vi "HexStringToBoolean.vi"(1 "Hex String":string) -> (0 "Boolean":bool)   [LabVIEW 2023]
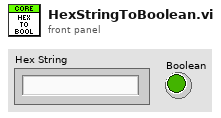
[diagram p1: front panel]
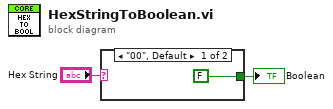
[diagram p0: block diagram]
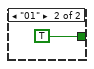
[diagram p2: hidden frame]
diagram:
  n1 = case shown="\"00\", Default" "Hex String" {
    tunnel: [FALSE ("Eco Wash") TRUE ("Eco Wash")] -> w1
    frame "00", Default {
    }
    frame "01" {
    }
  }
  "Boolean" <- w1
